vi "FakeTheoryWithControlsNotOnConnectorPane.vi"(9 "Input Data":string, 10 "Needle":string) -> (0 "error out":errorcluster)   [LabVIEW 2019, in "TheoryTest.lvlib" / "Support.lvlib"]
uses:
  Support.lvlib
  Assertion/Assertion.lvlib
panel:
  in  "Static Data (not on connector pane)":string="<static data>"
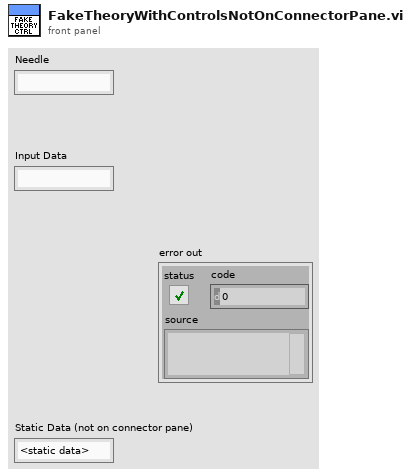
[diagram p1: front panel]
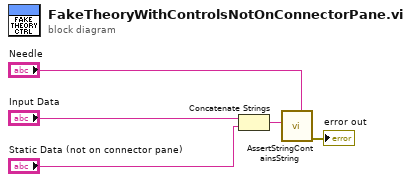
[diagram p0: block diagram]
diagram:
  n1 = Concatenate Strings("Input Data", "Static Data (not on connector pane)") -> (w3:string)
  n2 = call "AssertStringContainsString.vi"("Needle"="Needle", "Haystack"=w3) -> ("error out"=→"error out":errorcluster)  [unwired: 9 in]
